vi "Read_Multiple_TDMS_Data.vi"(10 "count (-1: all)":i64, 11 "offset (0)":i64) -> (0 "Vref1 @minMC":dbl, 1 "min Missing Codes":i32, 2 "Vref2 @minDNL":dbl, 3 "Vref1 @minDNL":dbl, 4 "Vref2 @minMC":dbl, 5 "min DNL":dbl)   [LabVIEW 2017]
uses:
  <vilib>/Utility/error.llb/DialogType.ctl
  Data_Analysis_Global_var.vi
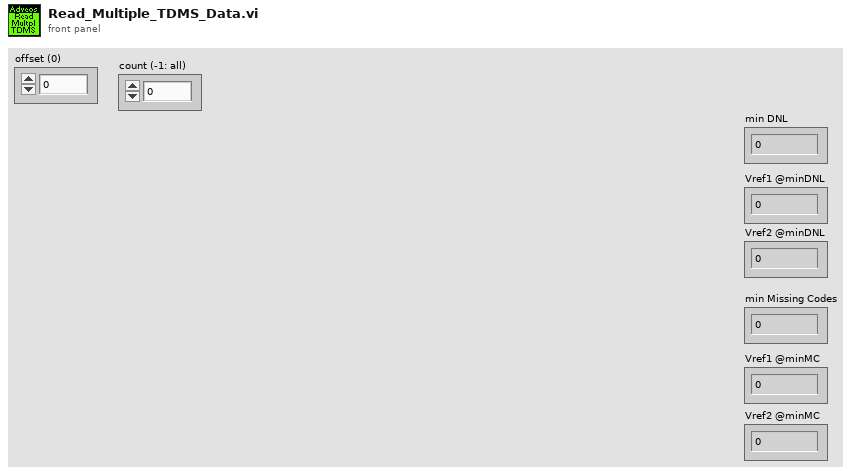
[diagram p1: front panel]
types:
  T1 = typedef "DialogType.ctl" = u16
  T2 = cluster{"unsigned byte array":i32[], "unsigned byte array":i32[]}
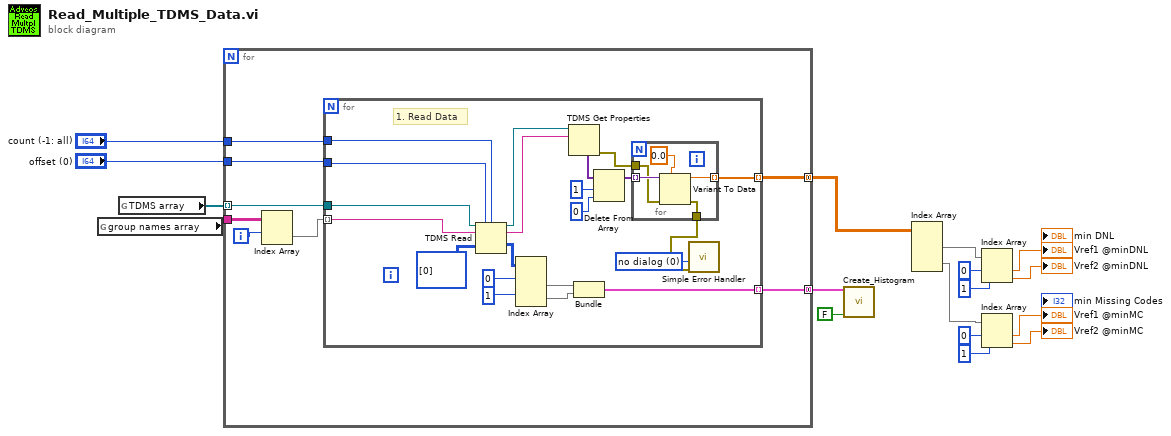
[diagram p0: block diagram]
diagram:
  n1 = global read "Data_Analysis_Global_var.vi" "group names array"() -> (w14:string[][])
  n2 = global read "Data_Analysis_Global_var.vi" "TDMS array"() -> (w15:refnum<k34>[])
  n3 = for {
    tunnel: "count (-1: all)" -> [w25]
    tunnel: "offset (0)" -> [w24]
    tunnel: w15 -> [w23] mode=indexing
    tunnel: w14 -> [w20]
    tunnel: [w22] -> w13 mode=concatenating
    tunnel: [w21] -> w12 mode=concatenating
    i -> [w19]
    n4 = Index Array(array=w20, index (row)=w19) -> (element=w18:string[])  [unwired: 1 in]
    n5 = for {
      tunnel: w25 -> [w42]
      tunnel: w24 -> [w41]
      tunnel: w23 -> [w40]
      tunnel: w18 -> [w26] mode=indexing
      tunnel: [w39] -> w22 mode=indexing
      tunnel: [w27] -> w21 mode=indexing
      w32 = T1 0 items=["no dialog", "OK message", "continue or stop message", "OK message + warnings", "continue/stop + warnings"] ("type of dialog (OK msg:1)")
      # "1. Read Data"
      n6 = TDMS Read(0:w40, 1:w41, 2:w42, 5:w26, 12:i32[][] [[0]] ("unsigned byte array")) -> (4:w29:refnum<k34>, 6:w28:string, 10:w43:i32[][])  [unwired: 3 in, 3 out]
      n7 = Index Array(array=w43, index (row) #1=0 ("index (row)"), index (row) #2=1 ("index (row)")) -> (element #1=w38:i32[], element #2=w37:i32[])  [unwired: 2 in]
      n8 = TDMS Get Properties(10:w28, 11:w29) -> (0:w35:errorcluster, 4:w34:variant[])  [unwired: 2 in, 6 out]
      n9 = Bundle("unsigned byte array"=w38, "unsigned byte array"=w37) -> (w39:T2)  [unwired: 1 in]
      n10 = Delete From Array(array=w34, length=1, index=0 ("length")) -> (array with subset deleted=w33:variant[])  [unwired: 1 out]
      n11 = for {
        tunnel: [w51] -> w27 mode=indexing
        tunnel: w33 -> [w50] mode=indexing
        tunnel: [w48] -> w36
        tunnel: w35 -> [w47]
        n12 = Variant To Data(error in=w47, type=0.0, Variant=w50) -> (data=w51:dbl, error out=w48:errorcluster)
      }
      n13 = call <vilib>:"Simple Error Handler.vi"("type of dialog (OK msg:1)"=w32, "error in (no error)"=w36) -> ()  [unwired: 3 in, 5 out]
    }
  }
  n14 = call "Create_Histogram.vi"("Average?"=FALSE, "XY Graph"=w13) -> ()  [unwired: 7 in, 3 out]
  n15 = Index Array(array=w12) -> (element #1=w11:dbl[], element #2=w1:dbl[])  [unwired: 4 in]
  n16 = Index Array(array=w11, index #1=0 ("index"), index #2=1 ("index")) -> (element #1=→"Vref1 @minDNL":dbl, element #2=→"Vref2 @minDNL":dbl)
  n17 = Index Array(array=w1, index #1=0 ("index"), index #2=1 ("index")) -> (element #1=→"Vref1 @minMC":dbl, element #2=→"Vref2 @minMC":dbl)
